vi "Use Index File.vi"(8 "error in":errorcluster, 10 "Index file":string="index.txt", 11 "Folder Path":path) -> (0 "error out":errorcluster, 2 "Index":i32)   [LabVIEW 2024]
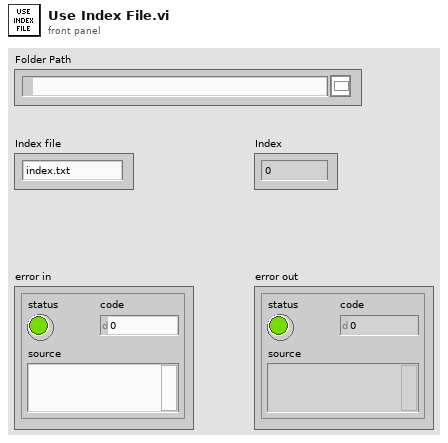
[diagram p1: front panel]
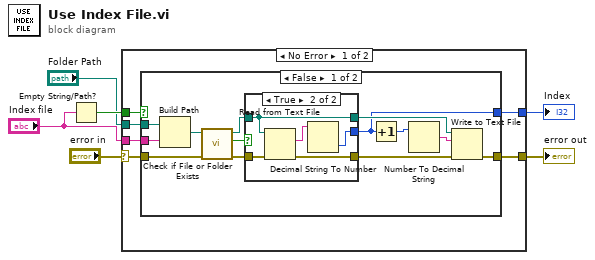
[diagram p0: block diagram]
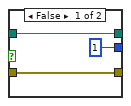
[diagram p2: hidden frame]
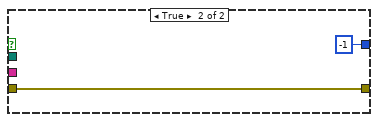
[diagram p3: hidden frame]
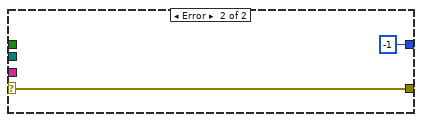
[diagram p4: hidden frame]
diagram:
  n1 = Empty String/Path?(string/path="Index file") -> (empty?=w5:bool)
  n2 = case shown="No Error" "error in" {
    selector: "error in" -> [w11 w37]
    tunnel: w5 -> [w12 _]
    tunnel: [w10 w37] -> w4
    tunnel: "Folder Path" -> [w9 _]
    tunnel: "Index file" -> [w8 _]
    tunnel: [w7 -1] -> w1
    frame No Error {
      n3 = case shown="False" w12 {
        tunnel: w11 -> [w22 w35]
        tunnel: [w14 w35] -> w10
        tunnel: w9 -> [w25 _]
        tunnel: w8 -> [w24 _]
        tunnel: [w13 -1] -> w7
        frame False {
          n4 = Build Path(base path=w25, name or relative path=w24) -> (appended path=w23:path)
          n5 = call <vilib>:"Check if File or Folder Exists.vi"("error in (no error)"=w22, "path"=w23) -> ("error out"=w20:errorcluster, "file or folder exists?"=w21:bool, "dup path"=w19:path)  [unwired: 7 in]
          n6 = case shown="True" w21 {
            tunnel: w20 -> [w27 w33]
            tunnel: w19 -> [w26 w29]
            tunnel: [1 w31] -> w13
            tunnel: [w27 w30] -> w18
            tunnel: [w26 w29] -> w17
            frame False {
            }
            frame True {
              n7 = Read from Text File(file (use dialog)=w29, error in=w33) -> (text=w32:string, error out=w30:errorcluster)  [unwired: 2 in, 2 out]
              n8 = Decimal String To Number(string=w32) -> (number=w31:i32)  [unwired: 2 in, 1 out]
            }
          }
          n9 = Increment(x=w13) -> (x+1=w16:i32)
          n10 = Number To Decimal String(number=w16) -> (decimal integer string=w15:string)  [unwired: 1 in]
          n11 = Write to Text File(file (use dialog)=w17, text=w15, error in=w18) -> (error out=w14:errorcluster)  [unwired: 1 in, 2 out]
        }
        frame True {
        }
      }
    }
    frame Error {
    }
  }
  "error out" <- w4
  "Index" <- w1
